vi "TortoiseGit Show Log.vi"(6 "Variant in":variant, 7 "Shift Pressed?":bool, 8 "error in (no error)":errorcluster, 10 "QD Combo Box Ref":refnum<vi>, 11 "QD Launch VI Ref":refnum<vi>) -> (0 "error out":errorcluster, 4 "Variant out":variant)   [LabVIEW 2018, in "TortoiseGit Show Log.lvlib"]
doc: "This plugin brings up the TortoiseGit log for the selected element.\n\nArguments: \n <nothing>, file = this VI\n folder, f, <shift modifier> = folder of VI on disk\n repo, r = repo containing VI\n class, c = folder of class containing VI\n library, l = folder of library containing VI\n project, p = folder of project of VI\n\nDefault Shortcut - [G]"
uses:
  TortoiseGit Show Log/TortoiseGit Show Log.lvlib
panel:
  in  "Undo Name":string
  # "Do not change the connector pane of this VI.\n\nSee the block diagram for directions on how to use this template."
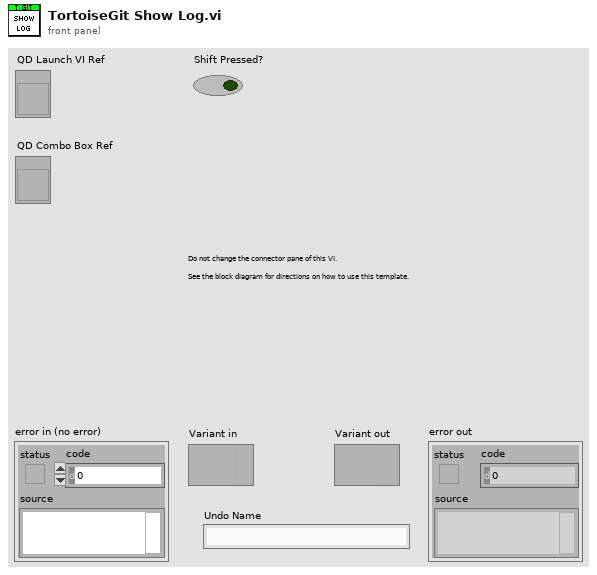
[diagram p1: front panel]
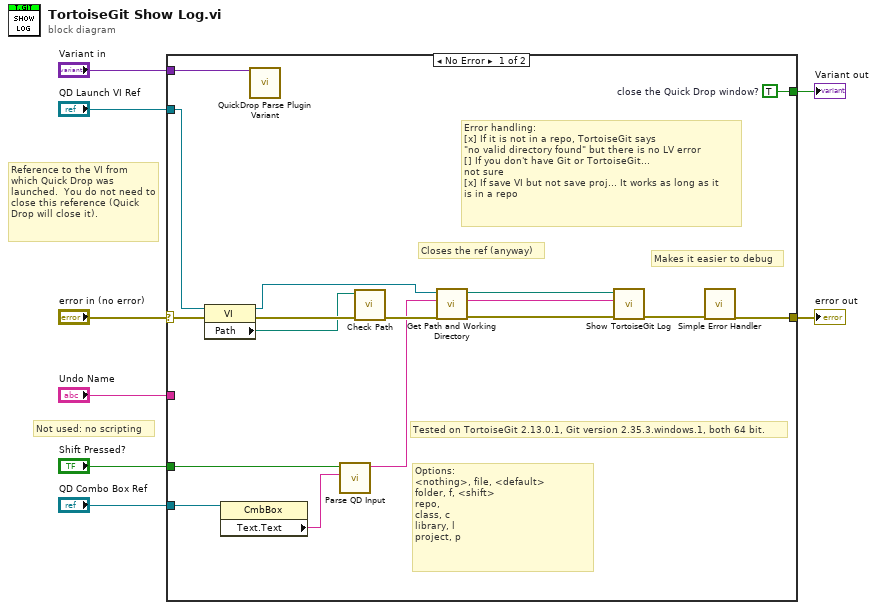
[diagram p0: block diagram]
diagram:
  # "Not used: no scripting"
  # "Reference to the VI from which Quick Drop was launched.  You do not need to close this reference (Quick Drop will close it)."
  n1 = case shown="No Error" "error in (no error)" {
    selector: "error in (no error)" -> [w24 w26]
    tunnel: [w21 w26] -> w7
    tunnel: "QD Launch VI Ref" -> [w23 _]
    tunnel: "QD Combo Box Ref" -> [w19 _]
    tunnel: "Variant in" -> [w25 _]
    tunnel: "Undo Name" -> [_ _]
    tunnel: [w22 _] -> w3
    tunnel: "Shift Pressed?" -> [w10 _]
    frame No Error {
      w22 = TRUE  # close the Quick Drop window?
      # "Makes it easier to debug"
      # "Tested on TortoiseGit 2.13.0.1, Git version 2.35.3.windows.1, both 64 bit."
      # "Options:\n<nothing>, file, <default>\nfolder, f, <shift>\nrepo, \nclass, c\nlibrary, l\nproject, p"
      # "Error handling:\n[x] If it is not in a repo, TortoiseGit says \n\"no valid directory found\" but there is no LV error\n[] If you don't have Git or TortoiseGit...\nnot sure\n[x] If save VI but not save proj... It works as long as it \nis in a repo"
      # "Closes the ref (anyway)"
      n2 = property class="VI"(reference=w23, error in=w24) -> (reference out=w17:refnum<vi>, error out=w18:errorcluster, "Path"=w15:path)
      n3 = property class="CmbBox"(reference=w19) -> ("Text.Text"=w11:string)  [unwired: 1 in, 2 out]
      n4 = call <vilib>:"QuickDrop Parse Plugin Variant.vi"("QDKS Variant in"=w25) -> ()  [unwired: 12 in, 3 out]
      n5 = call "Parse QD Input.vi"("QD window text"=w11, "Shift Pressed?"=w10) -> ("Element to show log for"=w9:string)  [unwired: 9 in]
      n6 = call "Check Path.vi"("error in"=w18, "Path"=w15) -> ("error out"=w16:errorcluster)  [unwired: 9 in]
      n7 = call "Get Path and Working Directory.vi"("error in"=w16, "Element to show log for"=w9, "VI in"=w17) -> ("error out"=w13:errorcluster, "/path value"=w14:string, "Working Directory"=w12:path)  [unwired: 6 in]
      n8 = call "Show TortoiseGit Log.vi"("error in"=w13, "/path value"=w14, "Working Directory"=w12) -> ("error out"=w20:errorcluster)  [unwired: 8 in]
      n9 = call <vilib>:"Simple Error Handler.vi"("error in (no error)"=w20) -> ("error out"=w21:errorcluster)  [unwired: 4 in, 4 out]
    }
    frame Error {
    }
  }
  "error out" <- w7
  "Variant out" <- w3
